vi "Test Overlays.vi"() -> ()   [LabVIEW 2020, in "VolatusConfig.lvlib"]
uses:
  VolatusConfig.lvlib
  lv-cdm/CDM-Config/Config-JSON/Config-JSON.lvclass
  lv-cdm/CDM-Config/Config Storage/Config Storage.lvclass
  C:/dev/lv20CE/relink/lv-cdm/CDM-Config/Config Storage/Config Storage.lvclass
  C:/dev/lv20CE/relink/lv-cdm/CDM-Config/Config-JSON/Config-JSON.lvclass
panel:
  in  "Path":path
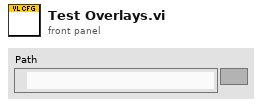
[diagram p1: front panel]
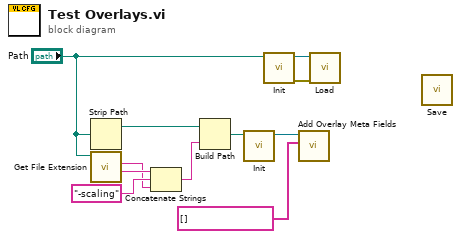
[diagram p0: block diagram]
diagram:
  n1 = Strip Path(path="Path") -> (stripped path=w5:path)  [unwired: 1 out]
  n2 = call <vilib>:"Get File Extension.vi"("file"="Path") -> ("filename without extension"=w8:string, "lowercase file extension"=w6:string)  [unwired: 6 in, 3 out]
  n3 = Concatenate Strings(w8, "-scaling" ("string"), w6) -> (w4:string)
  n4 = Build Path(base path=w5, name or relative path=w4) -> (appended path=w3:path)
  n5 = call "Init.vi"("Path"=w3) -> ("Config-JSON out"=w2:refnum<class "Config-JSON.lvclass">)  [unwired: 9 in, 1 out]
  n6 = call "Init.vi"("Path"="Path") -> ("error out"=w10:errorcluster, "Config-JSON out"=w11:refnum<class "Config-JSON.lvclass">)  [unwired: 9 in]
  n7 = call "Add Overlay Meta Fields.vi"("Meta Fields"=string[] [], "Config Storage in"=w2) -> ()  [unwired: 8 in, 2 out]
  n8 = call "Load.vi"("error in (no error)"=w10, "Config Storage in"=w11) -> ()  [unwired: 7 in, 3 out]
  n9 = call "Save.vi"() -> ()  [unwired: 10 in, 2 out]
